vi "gragh3.vi"() -> ()   [LabVIEW 2019]
panel:
  out "Waveform Chart":cluster{dbl, "number: 0 to 1":dbl}(graph)
  in  "stop":bool
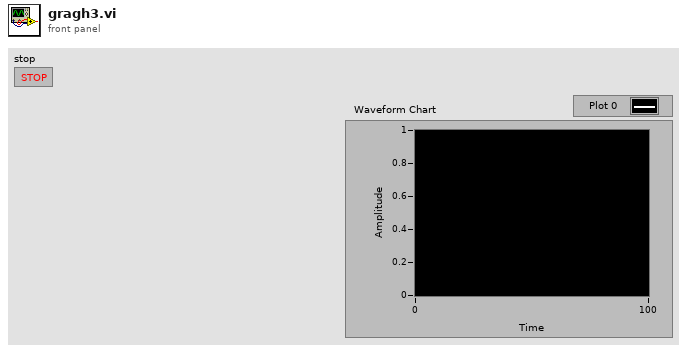
[diagram p1: front panel]
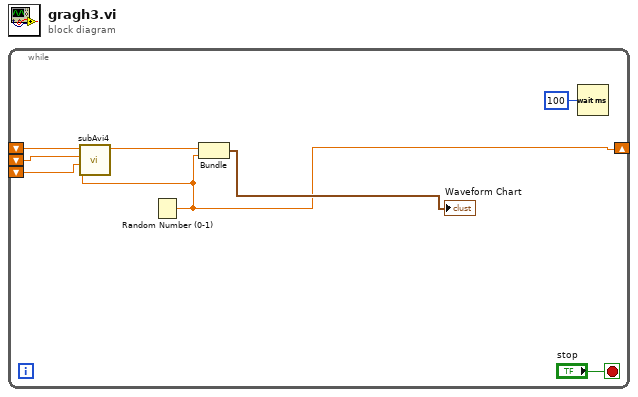
[diagram p0: block diagram]
diagram:
  n1 = while {
    shift-right: [w2] -> _
    shift-left: _ -> [w5]
    shift-left: _ -> [w4]
    shift-left: _ -> [w3]
    stop <- "stop" stop-if-true
    n2 = Random Number (0-1)() -> (number: 0 to 1=w2:dbl)
    n3 = call "subAvi4.vi"("Numeric 4"=w2, "Numeric 3"=w3, "Numeric 2"=w4, "Numeric"=w5) -> ("res"=w1:dbl)  [unwired: 7 in]
    n4 = Bundle("res"=w1, "number: 0 to 1"=w2) -> (→"Waveform Chart":cluster{"res":dbl, "number: 0 to 1":dbl})  [unwired: 1 in]
    n5 = Wait (ms)(milliseconds to wait=u32 100) -> ()  [unwired: 1 out]
  }
